vi "fix clfn scripting.vi"   [LabVIEW 2026]
uses:
  <vilib>/Utility/traverseref.llb/TRef TravTarget.ctl
  <vilib>/Utility/traverseref.llb/VI Scripting - Traverse.lvlib
types:
  T1 = typedef "TRef TravTarget.ctl" = enum16{"FP", "BD", "Other"}
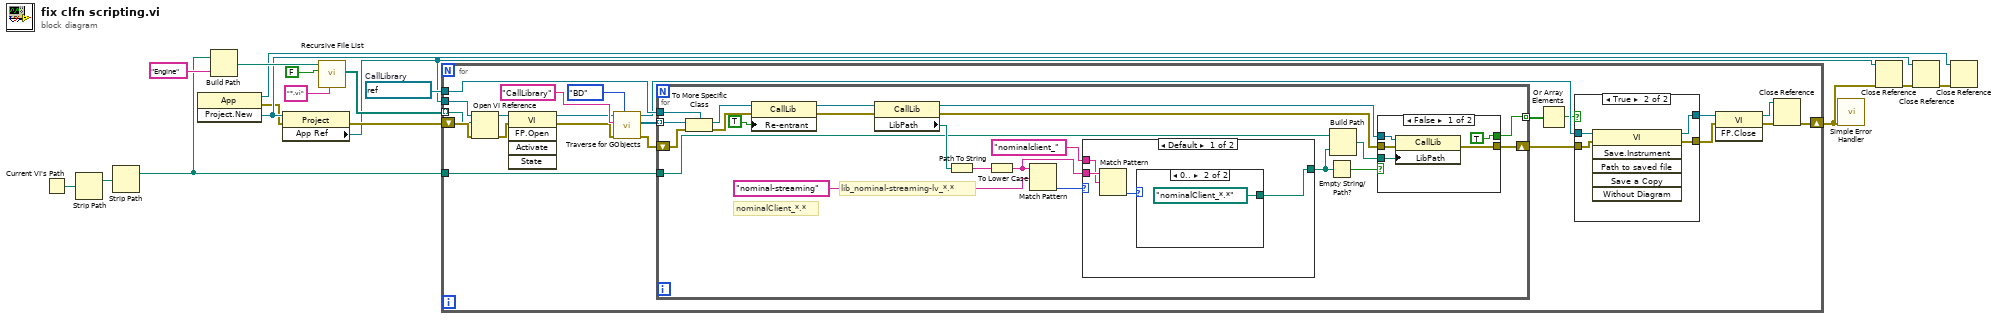
[diagram p0: block diagram]
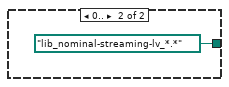
[diagram p5: hidden frame]
diagram:
  w17 = refnum<vi> refnum  # CallLibrary
  n1 = Current VI's Path() -> (path=w14:path)
  n2 = Strip Path(path=w14) -> (stripped path=w13:path)  [unwired: 1 out]
  n3 = Strip Path(path=w13) -> (stripped path=w1:path)  [unwired: 1 out]
  n4 = invoke class="App" method="Project.New"() -> (reference out=w8:refnum<vi>, error out=w5:errorcluster, "Project:New"=w6:refnum<vi>)  [unwired: 3 in]
  n5 = Build Path(base path=w1, name or relative path="Engine" ("Type")) -> (appended path=w11:path)
  n6 = property class="Project"(reference=w6, error in=w5) -> (error out=w4:errorcluster, "App Ref"=w2:refnum<vi>)  [unwired: 1 out]
  n7 = call <vilib>:"Recursive File List.vi"("pattern"="*.vi", "Treat LLBs as Folders?"=FALSE, "Folder Path"=w11) -> ("All Files in Dir"=w7:path[])  [unwired: 4 in, 4 out]
  n8 = for {
    tunnel: w17 -> [w36]
    shift-right: [w22] -> w15
    shift-left: w4 -> [w35]
    tunnel: w7 -> [w29] mode=indexing
    tunnel: w2 -> [w30]
    tunnel: w1 -> [w18]
    n9 = Open VI Reference(application reference (local)=w30, vi path=w29, error in (no error)=w35) -> (vi reference=w26:refnum<vi>, error out=w31:errorcluster)  [unwired: 3 in]
    n10 = invoke class="VI" method="FP.Open"(reference=w26, error in=w31) -> (reference out=w25:refnum<vi>, error out=w27:errorcluster)  [unwired: 3 in, 3 out]
    n11 = call <vilib>:"Traverse for GObjects.vi"("Traverse Target"=TRef_TravTarget."BD", "error in (no error)"=w27, "Class Name"="CallLibrary", "VI Refnum"=w25) -> ("error out"=w34:errorcluster, "References"=w37:refnum<vi>[], "dup VI Refnum"=w28:refnum<vi>)  [unwired: 4 in, 1 out]
    n12 = for {
      tunnel: w37 -> [w67] mode=indexing
      tunnel: w36 -> [w66]
      shift-right: [w60] -> w33
      shift-left: w34 -> [w63]
      tunnel: [w49] -> w20 mode=indexing
      tunnel: w18 -> [w48]
      # "nominalClient_*.*"
      # "lib_nominal-streaming-lv_*.*"
      n13 = To More Specific Class(target class=w66, reference=w67, error in=w63) -> (specific class reference=w65:refnum<vi>, error out=w62:errorcluster)
      n14 = property class="CallLib"(reference=w65, error in=w62, "Re-entrant"=TRUE ("Any Thread?")) -> (reference out=w58:refnum<vi>, error out=w61:errorcluster)
      n15 = property class="CallLib"(reference=w58, error in=w61) -> (reference out=w57:refnum<vi>, error out=w59:errorcluster, "LibPath"=w56:path)
      n16 = Path To String(path=w56) -> (string=w55:string)
      n17 = To Lower Case(string=w55) -> (all lower case string=w52:string)
      n18 = Match Pattern(string=w52, regular expression="nominal-streaming") -> (offset past match=w53:i32)  [unwired: 1 in, 3 out]
      n19 = case shown="Default" w53 {
        tunnel: w52 -> [w77 _]
        tunnel: "nominalclient_" -> [w76 _]
        tunnel: [w74 path "lib_nominal-streaming-lv_*.*" ("Library Path")] -> w47
        frame Default {
          n20 = Match Pattern(string=w77, regular expression=w76) -> (offset past match=w75:i32)  [unwired: 1 in, 3 out]
          n21 = case shown="0.." w75 {
            tunnel: [_ path "nominalClient_*.*"] -> w74
            frame Default {
            }
            frame 0.. {
            }
          }
        }
        frame 0.. {
        }
      }
      n22 = Empty String/Path?(string/path=w47) -> (empty?=w50:bool)
      n23 = Build Path(base path=w48, name or relative path=w47) -> (appended path=w46:path)
      n24 = case shown="False" w50 {
        tunnel: [w72 w73] -> w60
        tunnel: w59 -> [w71 w73]
        tunnel: w57 -> [w70 _]
        tunnel: [TRUE _] -> w49
        tunnel: w46 -> [w68 _]
        frame False {
          n25 = property class="CallLib"(reference=w70, error in=w71, "LibPath"=w68) -> (error out=w72:errorcluster)  [unwired: 1 out]
        }
        frame True {
        }
      }
    }
    n26 = Or Array Elements(Boolean array=w20) -> (logical OR=w19:bool)
    n27 = case shown="True" w19 {
      tunnel: w33 -> [w40 w45]
      tunnel: [w40 w44] -> w32
      tunnel: w28 -> [w41 w43]
      tunnel: [w41 w42] -> w23
      frame False {
      }
      frame True {
        n28 = invoke class="VI" method="Save.Instrument"(reference=w43, error in=w45) -> (reference out=w42:refnum<vi>, error out=w44:errorcluster)  [unwired: 4 in, 4 out]
      }
    }
    n29 = invoke class="VI" method="FP.Close"(reference=w23, error in=w32) -> (reference out=w21:refnum<vi>, error out=w24:errorcluster)  [unwired: 1 in, 1 out]
    n30 = Close Reference(reference=w21, error in (no error)=w24) -> (error out=w22:errorcluster)
  }
  n31 = call <vilib>:"Simple Error Handler.vi"("error in (no error)"=w15) -> ()  [unwired: 4 in, 5 out]
  n32 = Close Reference(reference=w2, error in (no error)=w15) -> (error out=w3:errorcluster)
  n33 = Close Reference(reference=w6, error in (no error)=w3) -> (error out=w16:errorcluster)
  n34 = Close Reference(reference=w8, error in (no error)=w16) -> ()  [unwired: 1 out]
